vi "SLSC Parse Capabilities File.vi"(8 "error in":errorcluster, 11 "module capabilities JSON string":string) -> (0 "error out":errorcluster, 3 "SLSC EDS module":T1)   [LabVIEW 2017]
doc: "This SLSC capabilities string parser deserializes a module's JSON capabilities string as read using SLSC Read NVMEM.vi example (*.bin)) and converts it to a cluster."
uses:
  EDSjsonStructure.ctl
  enum.ctl
  property.ctl
  command.ctl
  scale.ctl
  physicalChannel.ctl
  register.ctl
  <vilib>/addons/_JKI.lib/Serialization/JSON/JKI JSON Serialization.lvlib
panel:
  out "result string":string
  # "not working\nregisterMap->registers->initialValue"
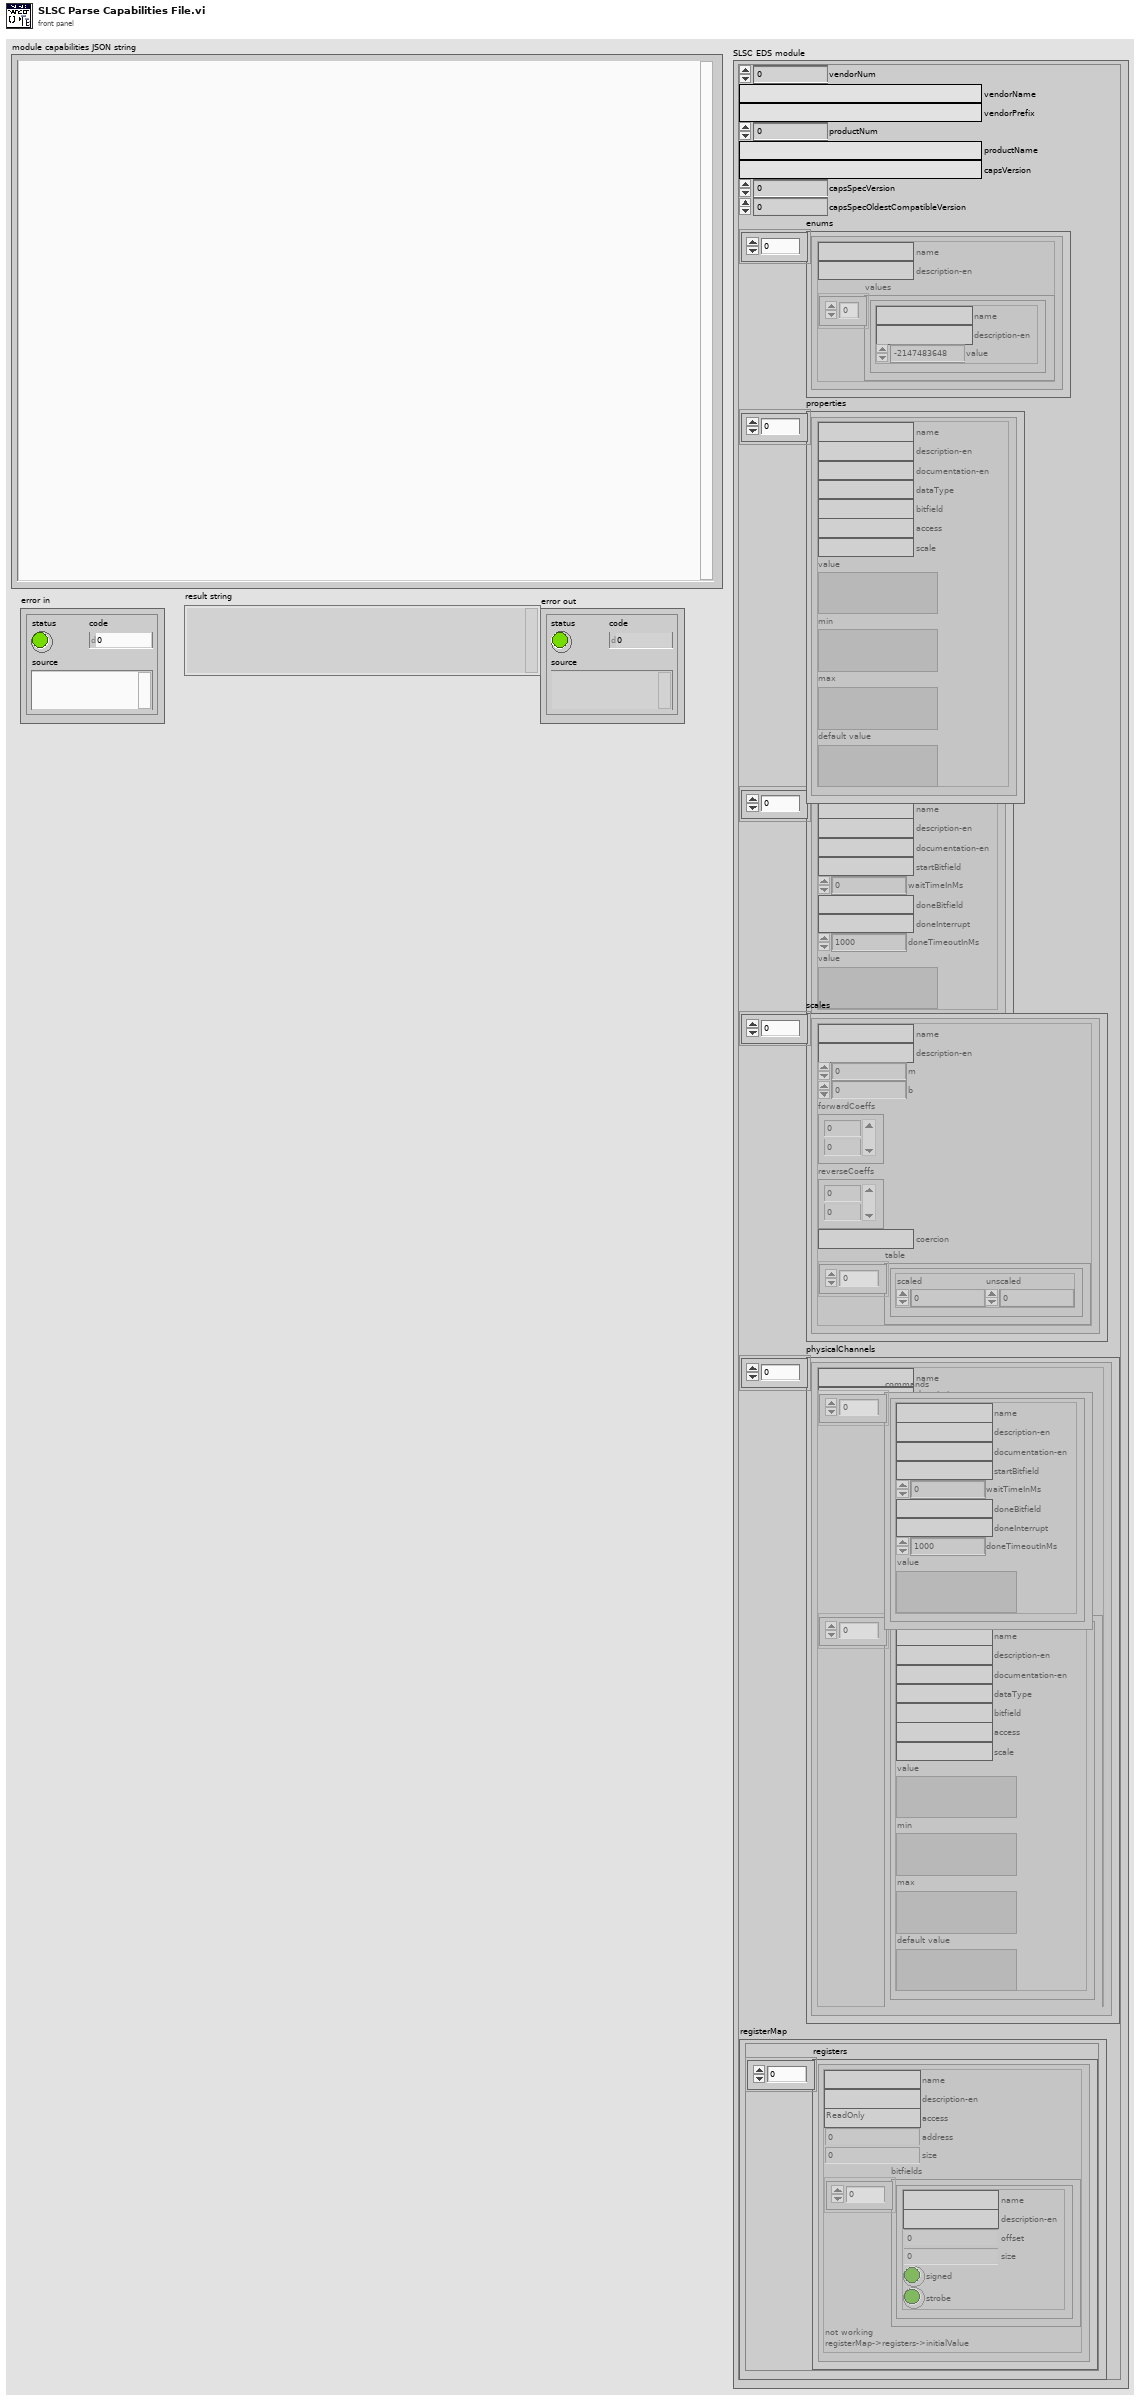
[diagram p1: front panel]
types:
  T1 = typedef "EDSjsonStructure.ctl" = cluster{"vendorNum":u32, "vendorName":string, "vendorPrefix":string, "productNum":u32, "productName":string, "capsVersion":string, "capsSpecVersion":u32, "capsSpecOldestCompatibleVersion":u32, "enums":T2[], "properties":T3[], "commands":T4[], "scales":T5[], "physicalChannels":T6[], "registerMap":cluster{"registers":T7[]}}
  T2 = typedef "enum.ctl" = cluster{"name":string, "description-en":string, "values":cluster{"name":string, "description-en":string, "value":i32}[]}
  T3 = typedef "property.ctl" = cluster{"name":string, "description-en":string, "documentation-en":string, "dataType":string, "bitfield":string, "access":string, "scale":string, "value":variant, "min":variant, "max":variant, "default value":variant}
  T4 = typedef "command.ctl" = cluster{"name":string, "description-en":string, "documentation-en":string, "startBitfield":string, "waitTimeInMs":i32, "doneBitfield":string, "doneInterrupt":string, "doneTimeoutInMs":i32, "value":variant}
  T5 = typedef "scale.ctl" = cluster{"name":string, "description-en":string, "m":dbl, "b":dbl, "forwardCoeffs":dbl[], "reverseCoeffs":dbl[], "coercion":string, "table":cluster{"scaled":dbl, "unscaled":dbl}[]}
  T6 = typedef "physicalChannel.ctl" = cluster{"name":string, "description-en":string, "commands":T4[], "properties":T3[]}
  T7 = typedef "register.ctl" = cluster{"name":string, "description-en":string, "access":string, "address":u32, "size":u32, "bitfields":cluster{"name":string, "description-en":string, "offset":u32, "size":u32, "signed":bool, "strobe":bool}[]}
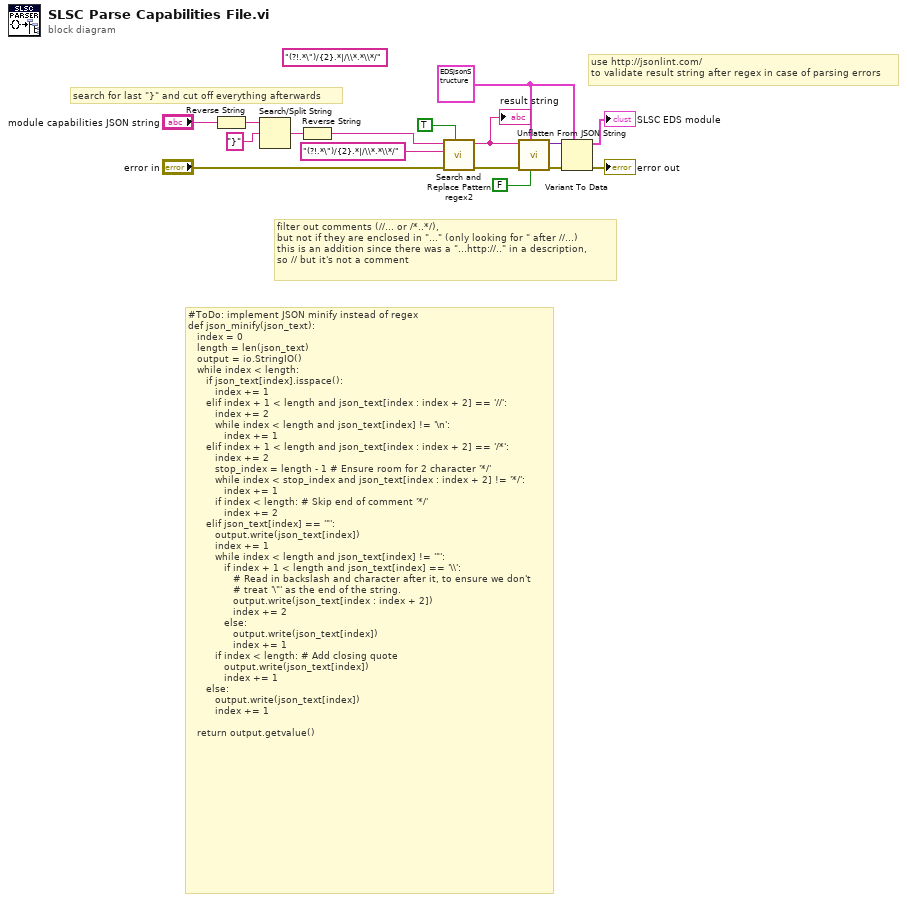
[diagram p0: block diagram]
diagram:
  (unwired) "(?!.*\")/{2}.*|/\\*.*\\*/" ("regular expression (\"\")")
  w10 = T1 {"vendorNum"=0, "vendorName"="", "vendorPrefix"="", "productNum"=0, "productName"="", "capsVersion"="", "capsSpecVersion"=0, "capsSpecOldestCompatibleVersion"=0, "enums"=[], "properties"=[], "commands"=[], "scales"=[], "physicalChannels"=[], "registerMap"={"registers"=[]}} ("ESDmoduleOptElements")
  # "#ToDo: implement JSON minify instead of regex\ndef json_minify(json_text):\n   index = 0\n   length = len(json_text)\n   output = io.StringIO()\n   while index < length:\n      if json_text[index].isspace():\n         index += 1\n      elif index + 1 < length and json_text[index : index + 2] == '//':\n         index += 2\n         while index < length and json_text[index] != '\\n':\n            index += 1\n      elif index + 1 < length and json_text[index : index + 2] == '/*':\n         index += 2\n         stop_index = length - 1 # Ensure room for 2 character '*/'\n         while index < stop_index and json_text[index : index + 2] != '*/':\n            index += 1\n         if index < length: # Skip end of comment '*/'\n            index += 2\n      elif json_text[index] == '\"':\n         output.write(json_text[index])\n         index += 1\n         while index < length and json_text[index] != '\"':\n            if index + 1 < length and json_text[index] == '\\\\':\n               # Read in backslash and character after it, to ensure we don't\n               # treat '\\\"' as the end of the string.\n               output.write(json_text[index : index + 2])\n               index += 2\n            else:\n               output.write(json_text[index])\n               index += 1\n         if index < length: # Add closing quote\n            output.write(json_text[index])\n            index += 1\n      else:\n         output.write(json_text[index])\n         index += 1\n\n   return output.getvalue()"
  # "search for last \"}\" and cut off everything afterwards"
  # "use http://jsonlint.com/\nto validate result string after regex in case of parsing errors"
  # "filter out comments (//... or /*..*/),\nbut not if they are enclosed in \"...\" (only looking for \" after //...)\nthis is an addition since there was a \"...http://..\" in a description, \nso // but it's not a comment"
  n1 = Reverse String(1:"module capabilities JSON string") -> (0:w4:string)
  n2 = Search/Split String(string=w4, search string/char (-)="}") -> (match + rest of string=w1:string)  [unwired: 1 in, 2 out]
  n3 = Reverse String(1:w1) -> (0:w2:string)
  n4 = call "Search and Replace Pattern regex2.vi"("replace all? (F)"=TRUE, "error in"="error in", "regular expression (\"\")"="(?!.*\")/{2}.*|/\\*.*\\*/" ("regular expression (\"\")"), "string"=w2) -> ("error out"=w8:errorcluster, "result string"=w14:string)  [unwired: 5 in, 1 out]
  "result string" <- w14
  n5 = call <vilib>:"Unflatten From JSON String.vi"("Nulls as Defaults (F)"=FALSE, "Type and Defaults"=w10, "error in (no error)"=w8, "JSON String"=w14) -> ("error out"=w13:errorcluster, "Variant"=w12:variant)  [unwired: 6 in]
  n6 = Variant To Data(error in=w13, type=w10, Variant=w12) -> (data=→"SLSC EDS module":T1, error out=→"error out":errorcluster)
